vi "Zmiana ustawienia położenia startowego po zmianie rozmiaru mapy.vi"(10 "Położenie startowe in":cluster{"X [px]":i16, "Y [px]":i16}, 11 ">mapa z trasą robota>":picture) -> (2 "Położenie startowe out":cluster{"X [px]":i16, "Y [px]":i16}, 3 "image data":T1)   [LabVIEW 2012, in "Biblioteka moduł map v3.lvlib" / "Obsługa grafiki mapy.lvlib"]
uses:
  <vilib>/picture/picture.llb/imagedata.ctl
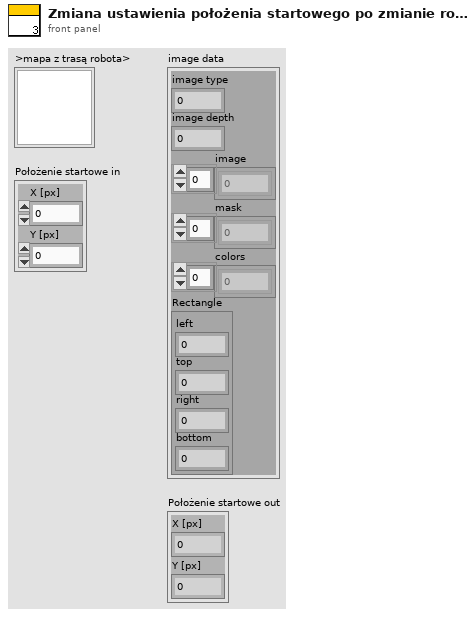
[diagram p1: front panel]
types:
  T1 = typedef "imagedata.ctl" = cluster{"image type":i32, "image depth":i32, "image":u8[], "mask":u8[], "colors":u32[], "Rectangle":cluster{"left":i16, "top":i16, "right":i16, "bottom":i16}}
  T2 = cluster{"left":i16, "top":i16, "right":i16, "bottom":i16}
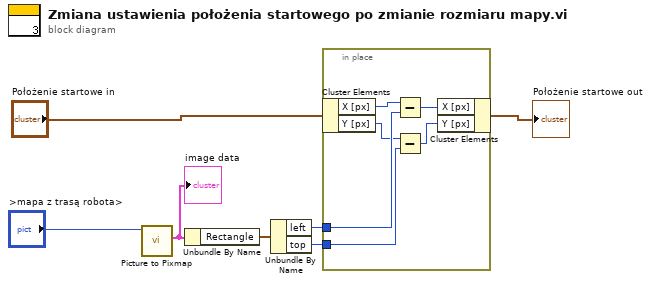
[diagram p0: block diagram]
diagram:
  n1 = call <vilib>:"Picture to Pixmap.vi"("picture"=">mapa z trasą robota>") -> ("image data"=w2:T1)  [unwired: 9 in, 1 out]
  "image data" <- w2
  n2 = Unbundle By Name(w2) -> ("Rectangle"=w3:T2)
  n3 = Unbundle By Name(w3) -> ("left"=w7:i16, "top"=w5:i16)
  n4 = in-place {
    in-place-border: w7 -> [w11]
    in-place-border: w5 -> [w10]
    n5 = in-place-cluster #1("Położenie startowe in") -> ("X [px]"=w13:i16, "Y [px]"=w9:i16)
    n6 = Subtract(x=w13, y=w11) -> (x-y=w12:i16)
    n7 = Subtract(x=w9, y=w10) -> (x-y=w8:i16)
    n8 = in-place-cluster #1("X [px]"=w12, "Y [px]"=w8) -> (→"Położenie startowe out":cluster{"X [px]":i16, "Y [px]":i16})
  }
